vi "Shift Register.vi"() -> ()   [LabVIEW 2022 SP3]
panel:
  out "Previous Iteration":u8
  out "Current Iteration":u8
  out "Numeric 2":u8
  in  "Numeric":u8
  in  "stop":bool
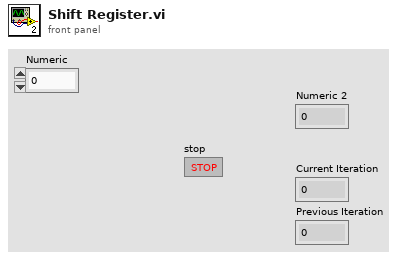
[diagram p1: front panel]
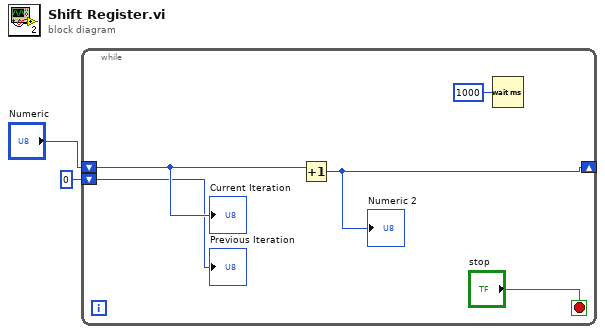
[diagram p0: block diagram]
diagram:
  n1 = while {
    shift-right: [w6] -> _
    shift-left: "Numeric" -> [w4]
    shift-left: u8 0 ("Numeric") -> [w3]
    stop <- "stop" stop-if-true
    n2 = Increment(x=w4) -> (x+1=w6:u8)
    "Numeric 2" <- w6
    n3 = Wait (ms)(milliseconds to wait=u32 1000) -> ()  [unwired: 1 out]
    "Current Iteration" <- w4
    "Previous Iteration" <- w3
  }
